vi "CursorLocation(Nanonis).vi"(4 "Setpoint":dbl=8.000000413701856e-11 format="%.0p", 5 "Value":dbl caption="Current Value" format="%#_2p", 6 "Position (Reframed)":cluster{"x (m)":dbl, "y (m)":dbl, "z (mm)":dbl} {"z (mm)" format="%.1f"; "y (m)" format="%.1p"; "x (m)" format="%.1p"}, 7 "Frame Properties (m)":T1) -> (0 "Cursor Size":cluster{"Width":i32, "Height":i32}, 1 "Current Above Setpoint?":bool=TRUE, 2 "Y-Coordinate":dbl, 3 "X-Coordinate":dbl)   [LabVIEW 2022 SP3]
doc: "Creates the XY position indicator on the image by scaling the data to fit the frame. Green light turns on when the Z-value is characteristic of being in the hole."
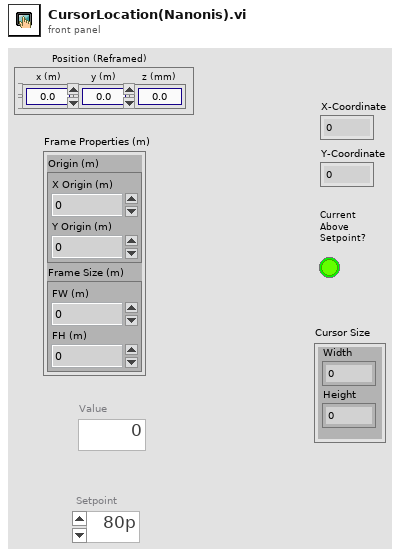
[diagram p1: front panel]
types:
  T1 = cluster{"Origin (m)":cluster{"X Origin (m)":dbl, "Y Origin (m)":dbl}, "Frame Size (m)":cluster{"FW (m)":dbl, "FH (m)":dbl}}
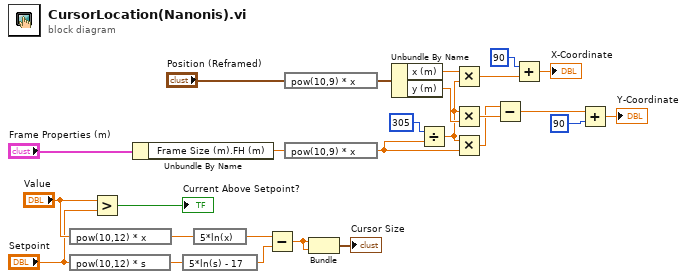
[diagram p0: block diagram]
diagram:
  n1 = expression code="pow(10,12) * x"("Value") -> (w8:dbl)
  n2 = expression code="pow(10,12) * s"("Setpoint") -> (w5:dbl)
  n3 = Greater?(x="Value", y="Setpoint") -> (0:→"Current Above Setpoint?":bool)
  n4 = Unbundle By Name("Frame Properties (m)") -> ("Frame Size (m).FH (m)"=w18:dbl)
  n5 = expression code="5*ln(s) - 17"(w5) -> (w4:dbl)
  n6 = expression code="5*ln(x)"(w8) -> (w3:dbl)
  n7 = Subtract(x=w3, y=w4) -> (x-y=w2:dbl)
  n8 = expression code="pow(10,9) * x"("Position (Reframed)") -> (w26:cluster{"x (m)":dbl, "y (m)":dbl, "z (mm)":dbl})
  n9 = expression code="pow(10,9) * x"(w18) -> (w14:dbl)
  n10 = Bundle(w2, w2) -> (→"Cursor Size":cluster{dbl, dbl})  [unwired: 1 in]
  n11 = Unbundle By Name(w26) -> ("x (m)"=w24:dbl, "y (m)"=w23:dbl)
  n12 = Divide(x=305, y=w14) -> (x/y=w16:dbl)
  n13 = Multiply(x=w24, y=w16) -> (x*y=w22:dbl)
  n14 = Multiply(x=w16, y=w23) -> (x*y=w19:dbl)
  n15 = Multiply(x=w16, y=w14) -> (x*y=w15:dbl)
  n16 = Subtract(x=w15, y=w19) -> (x-y=w12:dbl)
  n17 = Add(x=90, y=w22) -> (x+y=→"X-Coordinate":dbl)
  n18 = Add(x=w12, y=90) -> (x+y=→"Y-Coordinate":dbl)
